vi "Step Trigger VI.vi"() -> ()   [LabVIEW 2019, in "TimingDRV System Explorer.lvlib"]
uses:
  TimingDRV System Explorer.lvlib
  <vilib>/NI VeriStand/Execution/CustomDevice/NI VeriStand - Send Custom Device Message (String).vi
  <vilib>/NI VeriStand/Execution/CustomDevice/NI_VS Custom Device ExecutionAPI.lvlib
panel:
  out "Numeric":i32
  out "error out":errorcluster
  in  "Stop":bool
  in  "Send Message":bool
  out "String Response":string
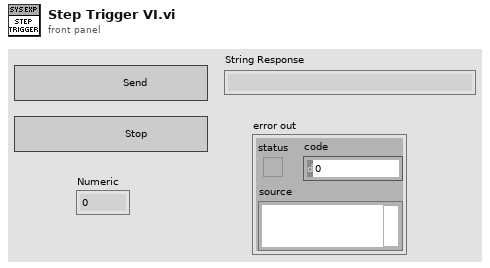
[diagram p1: front panel]
types:
  T1 = typedef "NI_VS Custom Device ExecutionAPI.lvlib/Custom Device Ref.ctl" = refnum<k24>
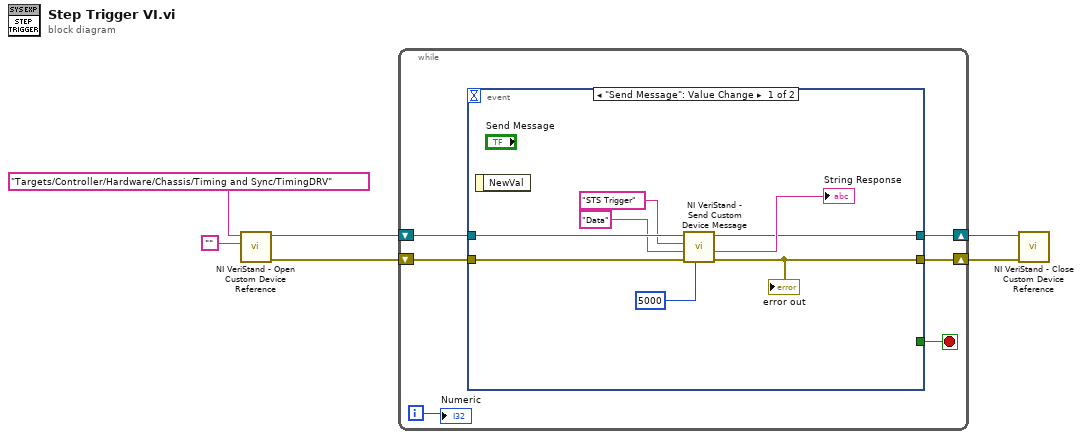
[diagram p0: block diagram]
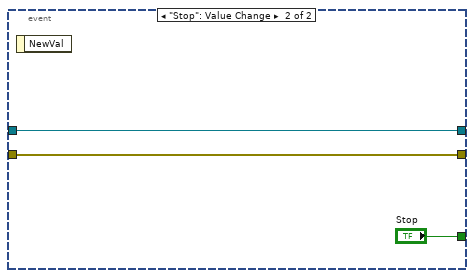
[diagram p2: hidden frame]
diagram:
  n1 = call <vilib>:"NI VeriStand - Open Custom Device Reference.vi"("Gateway IP Address (\"\": localhost)"="", "Custom Device Path"="Targets/Controller/Hardware/Chassis/Timing and Sync/TimingDRV") -> ("error out"=w4:errorcluster, "Custom Device"=w5:T1)  [unwired: 8 in]
  n2 = while {
    shift-right: [w9] -> w2
    shift-left: w5 -> [w12]
    shift-right: [w10] -> w3
    shift-left: w4 -> [w11]
    i -> [w7]
    stop <- w8 stop-if-true
    n3 = event shown="[0] \"Send Message\": Value Change" {
      selector: _ -> [_ _]
      dyn-events: _ -> [_ _]
      timeout: _ -> [_ _]
      tunnel: w12 -> [w19 w23]
      tunnel: w11 -> [w18 w22]
      tunnel: [w13 w22] -> w10
      tunnel: [w15 w23] -> w9
      tunnel: [_ "Stop"] -> w8
      event "Send Message": Value Change {
        n4 = event-data() -> ()  [unwired: 1 in, 1 out]
        n5 = call-poly <vilib>:"NI VeriStand - Send Custom Device Message.vi"("Timeout ms (5000)"=5000, "error in (no error)"=w18, "Data"="Data", "Command"="STS Trigger", "Custom Device in"=w19) -> ("error out"=w13:errorcluster, "Response"=→"String Response":string, "Custom Device out"=w15:T1)  [unwired: 4 in]
        "error out" <- w13
      }
      event "Stop": Value Change {
        n6 = event-data() -> ()  [unwired: 1 in, 1 out]
      }
    }
    "Numeric" <- w7
  }
  n7 = call <vilib>:"NI VeriStand - Close Custom Device Reference.vi"("error in (no error)"=w3, "Custom Device"=w2) -> ()  [unwired: 9 in, 1 out]
